vi "Read RawData.vi"(8 "error in (no error)":errorcluster, 9 "WCM":bool, 10 "# of scans":i32, 11 "UV-VIS in":refnum<class "CCD_camera.lvclass">) -> (0 "error out":errorcluster, 1 "Channel II OUT":sgl[][](array[numeric]), 2 "Channel I OUT":sgl[][](array[numeric]), 3 "UV-VIS out":refnum<class "CCD_camera.lvclass">, 4 "WCM_values OUT":sgl[](array[numeric]))   [LabVIEW 2015, in "CCD_camera.lvclass"]
uses:
  CCD_camera.lvclass
  dependecies/ControlsVIs/Clusters-def/Message types.ctl
  dependecies/ControlsVIs/Clusters-def/Standard Command.ctl
  dependecies/ControlsVIs/Clusters-def/OSc-WCM_max_value.ctl
  dependecies/Error Code Enum typedef.ctl
  Oscilloscope/Oscilloscope.lvclass
  Message/Message.lvclass
  GeneralFunctionality/GeneralFunctionality.lvclass
panel:
  in  "Booléen":bool
  out "error IO":errorcluster
  out "Graphe":i32[](graph)
  in  "Binning Horizontal":i32=1
  out "DLL error code":u32=20066
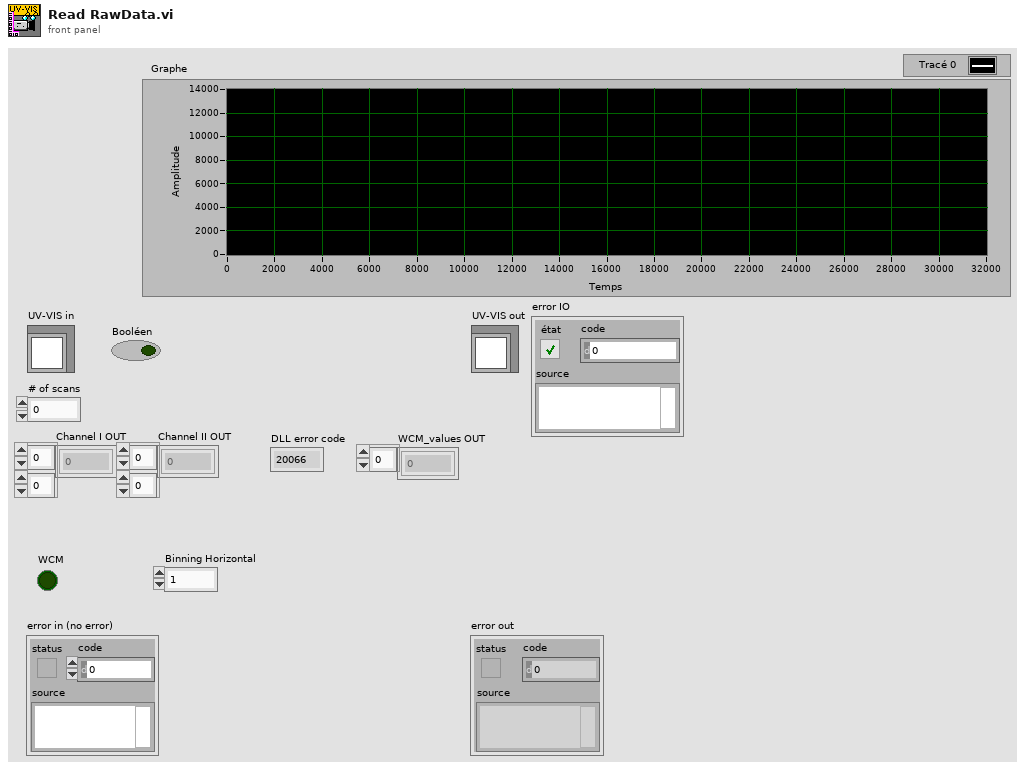
[diagram p1: front panel]
types:
  T1 = typedef "Message types.ctl" = string
  T2 = typedef "Standard Command.ctl" = cluster{"command":string, "data":variant}
  T3 = typedef "Oscilloscope.lvclass/OSc-WCM_max_value.ctl" = cluster{"WCM_max_value":dbl}
  T4 = typedef "Error Code Enum typedef.ctl" = enum32{"N/A (0)", "DRV_ERROR_CODES", "DRV_SUCCESS", "DRV_VXDNOTINSTALLED", "DRV_ERROR_SCAN", "DRV_ERROR_CHECK_SUM", "DRV_ERROR_FILELOAD", "DRV_UNKNOWN_FUNC", "DRV_ERROR_VXD_INIT", "DRV_ERROR_ADDRESS", "DRV_ERROR_PAGELOCK", "DRV_ERROR_PAGEUNLOCK", "DRV_ERROR_BOARDTEST", "DRV_ERROR_ACK", "DRV_ERROR_UP_FIFO", "DRV_ERROR_PATTERN", "N/A (16)", "DRV_ACQUISITION_ERRORS", "DRV_ACQ_BUFFER", "DRV_ACQ_DOWNFIFO_FULL", "DRV_PROC_UNKONWN_INSTRUCTION", "DRV_ILLEGAL_OP_CODE", "DRV_KINETIC_TIME_NOT_MET", "DRV_ACCUM_TIME_NOT_MET", "DRV_NO_NEW_DATA", "N/A (25)", "DRV_SPOOLERROR", "N/A (27)", "N/A (28)", "N/A (29)", "N/A (30)", "N/A (31)", "N/A (32)", "DRV_TEMPERATURE_CODES", "DRV_TEMPERATURE_OFF", "DRV_TEMPERATURE_NOT_STABILIZED", "DRV_TEMPERATURE_STABILIZED", "DRV_TEMPERATURE_NOT_REACHED", "DRV_TEMPERATURE_OUT_RANGE", "DRV_TEMPERATURE_NOT_SUPPORTED", "DRV_TEMPERATURE_DRIFT", "N/A (41)", "N/A (42)", "N/A (43)", "N/A (44)", "N/A (45)", "N/A (46)", "N/A (47)", "N/A (48)", "DRV_GENERAL_ERRORS", "DRV_INVALID_AUX", "DRV_COF_NOTLOADED", "DRV_FPGAPROG", "DRV_FLEXERROR", "DRV_GPIBERROR", "N/A (55)", "N/A (56)", "N/A (57)", "N/A (58)", "N/A (59)", "N/A (60)", "N/A (61)", "N/A (62)", "N/A (63)", "DRV_DATATYPE", "DRV_DRIVER_ERRORS", "DRV_P1INVALID", "DRV_P2INVALID", "DRV_P3INVALID", "DRV_P4INVALID", "DRV_INIERROR", "DRV_COFERROR", "DRV_ACQUIRING", "DRV_IDLE", "DRV_TEMPCYCLE", "DRV_NOT_INITIALIZED", "DRV_P5INVALID", "DRV_P6INVALID", "DRV_INVALID_MODE", "DRV_INVALID_FILTER", "DRV_I2CERRORS", "DRV_I2CDEVNOTFOUND", "DRV_I2CTIMEOUT", "DRV_P7INVALID", "N/A (84)", "N/A (85)", "N/A (86)", "N/A (87)", "N/A (88)", "N/A (89)", "DRV_IOCERROR", "DRV_VRMVERSIONERROR"}
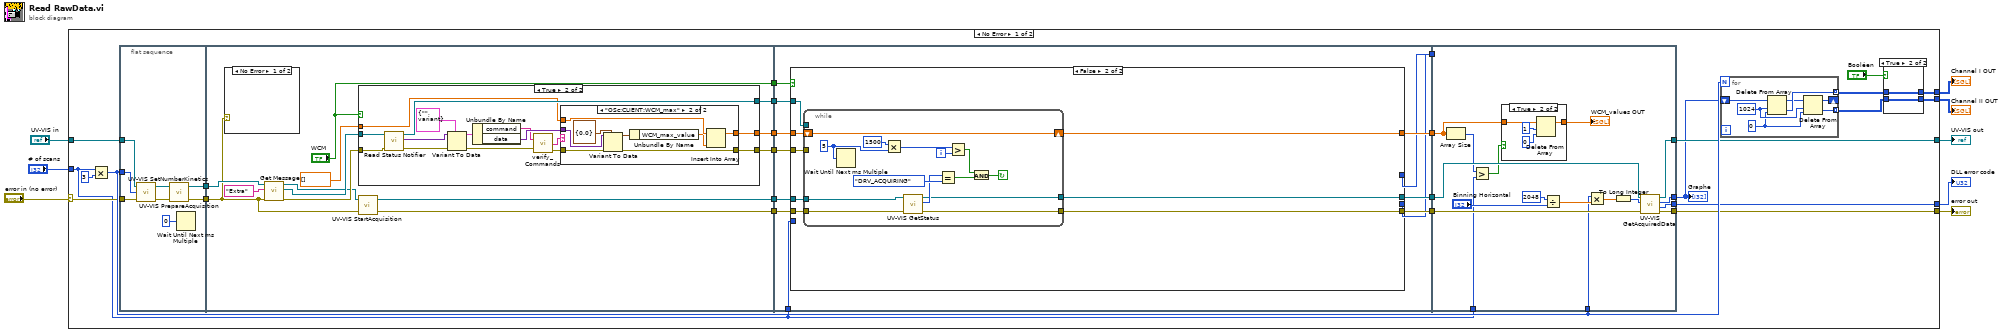
[diagram p0: block diagram]
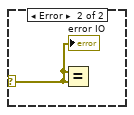
[diagram p3: hidden frame]
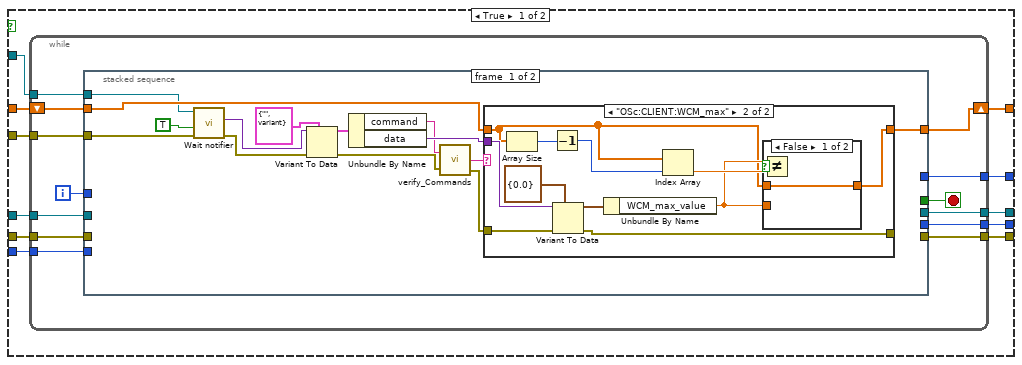
[diagram p6: hidden frame]
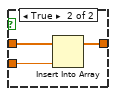
[diagram p8: hidden frame]
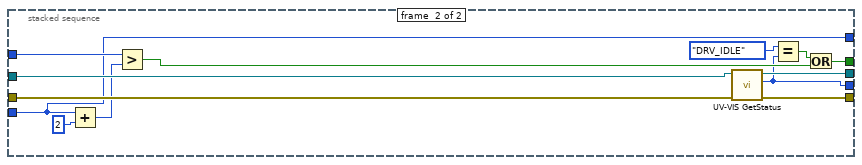
[diagram p9: hidden frame]
diagram:
  n1 = case shown="No Error" "error in (no error)" {
    selector: "error in (no error)" -> [w31 w223]
    tunnel: [w21 w223] -> w7
    tunnel: [w28 w222] -> w6
    tunnel: "UV-VIS in" -> [w30 w222]
    tunnel: "# of scans" -> [w16 _]
    tunnel: [w12 _] -> w3
    tunnel: [w11 _] -> w2
    tunnel: [w22 _] -> w1
    frame No Error {
      n2 = Multiply(x=w16, y=3) -> (x*y=w32:i32)
      n3 = flat-sequence {
        tunnel: [w52] -> w35
        tunnel: w32 -> [w51]
        tunnel: w30 -> [w49]
        tunnel: w31 -> [w50]
        tunnel: [w47] -> w29
        tunnel: w35 -> [w56]
        tunnel: [w67] -> w34
        tunnel: w29 -> [w65]
        tunnel: [w66] -> w27
        tunnel: ["WCM"] -> w24
        tunnel: [w61] -> w19
        tunnel: [w60] -> w18
        tunnel: [w59] -> w17
        tunnel: w34 -> [w108]
        tunnel: [w105] -> w26
        tunnel: w27 -> [w107]
        tunnel: [w106] -> w25
        tunnel: w24 -> [w100]
        tunnel: [w102] -> w23
        tunnel: w19 -> [w104]
        tunnel: w18 -> [w101]
        tunnel: w17 -> [w103]
        tunnel: w16 -> [w99]
        tunnel: [w98] -> w15
        tunnel: [w97] -> w14
        tunnel: w26 -> [w211]
        tunnel: w32 -> [w203]
        tunnel: w25 -> [w208]
        tunnel: [w215] -> w20
        tunnel: [w214] -> w22
        tunnel: [w209] -> w28
        tunnel: [w207] -> w21
        tunnel: w23 -> [w206]
        tunnel: w16 -> [w201]
        tunnel: w15 -> [_]
        tunnel: w14 -> [_]
        frame #0 {
          n4 = call "UV-VIS SetNumberKinetics.vi"("error in (no error)"=w50, "number"=w51, "Detector in"=w49) -> ("error out"=w54:errorcluster, "Detector out"=w48:refnum<class "CCD_camera.lvclass">)  [unwired: 1 out]
          n5 = call "UV-VIS PrepareAcquisition.vi"("error in (no error)"=w54, "Detector in"=w48) -> ("error out"=w52:errorcluster, "Detector out"=w47:refnum<class "CCD_camera.lvclass">)  [unwired: 1 in, 1 out]
          n6 = Wait Until Next ms Multiple(millisecond multiple=u32 0 ("n millisecondes")) -> ()  [unwired: 1 out]
        }
        frame #1 {
          n7 = case shown="No Error" w56 {
            selector: w56 -> [_ w68]
            frame No Error {
            }
            frame Error {
              n8 = Equal?(x=w68, y=w68) -> ()  [unwired: 1 out]
              "error IO" <- w68
            }
          }
          n9 = call "Get Message.vi"("error in (no error)"=w56, "Message type"=T1 "Extra", "GeneralFunctionality en entrée"=w65) -> ("error out"=w57:errorcluster, "Message.lvclass"=w58:refnum<class "Message.lvclass">, "GeneralFunctionality en sortie"=w55:refnum<class "CCD_camera.lvclass">)  [unwired: 6 in]
          n10 = case shown="True" "WCM" {
            tunnel: [w70 w72] -> w60
            tunnel: [w71 w86] -> w61
            tunnel: w58 -> [w71 w85]
            tunnel: w57 -> [w70 w81]
            tunnel: dbl[] [] -> [w69 w73]
            tunnel: [w69 w74] -> w59
            frame False {
            }
            frame True {
              n11 = call "Read Status Notifier.vi"("error in (no error)"=w81, "Message in"=w85) -> ("error out"=w80:errorcluster, "latest notification"=w82:variant, "Message out"=w86:refnum<class "Message.lvclass">)  [unwired: 6 in, 1 out]
              n12 = Variant To Data(error in=w80, type=T2 {"command"="", "data"=variant} ("input cluster"), Variant=w82) -> (data=w84:T2, error out=w75:errorcluster)
              n13 = Unbundle By Name(w84) -> ("command"=w76:string, "data"=w79:variant)
              n14 = call "verify_Commands.vi"("Command"=w76, "error in"=w75) -> ("Command out"=w77:string, "error out"=w78:errorcluster)  [unwired: 1 out]
              n15 = case shown="\"OSc:CLIENT:WCM_max\"" w77 {
                tunnel: w78 -> [w88 w96]
                tunnel: [w88 w94] -> w72
                tunnel: w79 -> [_ w95]
                tunnel: w73 -> [w87 w91]
                tunnel: [w87 w90] -> w74
                frame "Error", Default {
                }
                frame "OSc:CLIENT:WCM_max" {
                  n16 = Variant To Data(error in=w96, type=T3 {"WCM_max_value"=0.0} ("ELYSE pulses counter"), Variant=w95) -> (data=w92:T3, error out=w94:errorcluster)
                  n17 = Unbundle By Name(w92) -> ("WCM_max_value"=w89:dbl)
                  n18 = Insert Into Array(array=w91, new element=w89) -> (w90:dbl[])  [unwired: 1 in]
                }
              }
            }
          }
          n19 = call "UV-VIS StartAcquisition.vi"("error in (no error)"=w56, "Detector in"=w55) -> ("error out"=w67:errorcluster, "Detector out"=w66:refnum<class "CCD_camera.lvclass">)  [unwired: 1 in, 1 out]
        }
        frame #2 {
          n20 = case shown="False" w100 {
            tunnel: w108 -> [w119 w185]
            tunnel: w107 -> [w118 w184]
            tunnel: [w113 w183] -> w106
            tunnel: [w112 w182] -> w105
            tunnel: w104 -> [w117 w181]
            tunnel: w103 -> [w116 w180]
            tunnel: [w115 w179] -> w102
            tunnel: w101 -> [w114 w178]
            tunnel: w99 -> [w111 _]
            tunnel: [w110 _] -> w98
            tunnel: [w109 _] -> w97
            frame True {
              n21 = while {
                tunnel: w119 -> [w127]
                tunnel: w118 -> [w128]
                tunnel: w117 -> [w130]
                shift-right: [w131] -> w115
                shift-left: w116 -> [w132]
                tunnel: w114 -> [w129]
                tunnel: [w126] -> w113
                tunnel: [w125] -> w112
                tunnel: w111 -> [w122]
                tunnel: [w121] -> w110
                tunnel: [w120] -> w109
                i -> [w124]
                stop <- w123 stop-if-true
                n22 = stacked-sequence {
                  tunnel: w132 -> [w146 _]
                  tunnel: [w145 _] -> w131
                  tunnel: w130 -> [w137 _]
                  tunnel: w129 -> [w136 _]
                  tunnel: w128 -> [_ w177]
                  tunnel: w127 -> [_ w175]
                  tunnel: [_ w176] -> w126
                  tunnel: [_ w174] -> w125
                  tunnel: w124 -> [_ w170]
                  tunnel: [_ w169] -> w123
                  tunnel: w122 -> [_ w165]
                  tunnel: [_ w166] -> w121
                  tunnel: [_ w165] -> w120
                  frame #0 {
                    n23 = call "Wait notifier.vi"("error in (no error)"=w136, "ignorer les précédents (F)"=TRUE, "Message en entrée"=w137) -> ("error out"=w134:errorcluster, "notification"=w135:variant)  [unwired: 6 in, 1 out]
                    n24 = Variant To Data(error in=w134, type=T2 {"command"="", "data"=variant} ("input cluster"), Variant=w135) -> (data=w144:T2, error out=w138:errorcluster)
                    n25 = Unbundle By Name(w144) -> ("command"=w139:string, "data"=w142:variant)
                    n26 = call "verify_Commands.vi"("Command"=w139, "error in"=w138) -> ("Command out"=w140:string, "error out"=w141:errorcluster)  [unwired: 1 out]
                    n27 = case shown="\"OSc:CLIENT:WCM_max\"" w140 {
                      tunnel: w141 -> [w148 w160]
                      tunnel: [w148 w158] -> _
                      tunnel: w142 -> [_ w159]
                      tunnel: w146 -> [w147 w151]
                      tunnel: [w147 w155] -> w145
                      frame "Error", Default {
                      }
                      frame "OSc:CLIENT:WCM_max" {
                        n28 = Array Size(array=w151) -> (size(s)=w150:i32)
                        n29 = Decrement(x=w150) -> (x-1=w149:i32)
                        n30 = Variant To Data(error in=w160, type=T3 {"WCM_max_value"=0.0} ("ELYSE pulses counter"), Variant=w159) -> (data=w156:T3, error out=w158:errorcluster)
                        n31 = Unbundle By Name(w156) -> ("WCM_max_value"=w152:dbl)
                        n32 = Index Array(array=w151, index=w149) -> (element=w154:dbl)
                        n33 = Not Equal?(x=w152, y=w154) -> (x != y?=w153:bool)
                        n34 = case shown="False" w153 {
                          tunnel: w151 -> [w161 w164]
                          tunnel: [w161 w163] -> w155
                          tunnel: w152 -> [_ w162]
                          frame False {
                          }
                          frame True {
                            n35 = Insert Into Array(array=w164, new element=w162) -> (w163:dbl[])  [unwired: 1 in]
                          }
                        }
                      }
                    }
                  }
                  frame #1 {
                    n36 = Add(x=w165, y=2) -> (x+y=w168:i32)
                    n37 = Greater?(x=w170, y=w168) -> (0:w171:bool)
                    n38 = call "UV-VIS GetStatus.vi"("error in (no error)"=w175, "Detector in"=w177) -> ("error out"=w174:errorcluster, "status"=w166:T4, "Detector out"=w176:refnum<class "CCD_camera.lvclass">)  [unwired: 2 in, 1 out]
                    n39 = Equal?(x=Error_Code_Enum_typedef."DRV_IDLE" ("y"), y=w166) -> (x = y?=w172:bool)
                    n40 = Or(x=w172, y=w171) -> (x .or. y?=w169:bool)
                  }
                }
              }
            }
            frame False {
              n41 = while {
                tunnel: w185 -> [w197]
                tunnel: [w196] -> w182
                tunnel: w184 -> [w195]
                tunnel: [w194] -> w183
                tunnel: w181 -> [_]
                shift-right: [w186] -> w179
                shift-left: w180 -> [w186]
                tunnel: w178 -> [_]
                i -> [w187]
                stop <- w191 continue-if-true
                w189 = u32 5 ("n millisecondes")
                n42 = Wait Until Next ms Multiple(millisecond multiple=w189) -> ()  [unwired: 1 out]
                n43 = Multiply(x=1500 ("y"), y=w189) -> (x*y=w188:u32)
                n44 = call "UV-VIS GetStatus.vi"("error in (no error)"=w197, "Detector in"=w195) -> ("error out"=w196:errorcluster, "status"=w198:T4, "Detector out"=w194:refnum<class "CCD_camera.lvclass">)  [unwired: 2 in, 1 out]
                n45 = Equal?(x=w198, y=Error_Code_Enum_typedef."DRV_ACQUIRING") -> (x = y?=w193:bool)
                n46 = Greater?(x=w188, y=w187) -> (0:w192:bool)
                n47 = And(x=w192, y=w193) -> (x .and. y?=w191:bool)
              }
            }
          }
        }
        frame #3 {
          n48 = Array Size(array=w206) -> (size(s)=w204:i32)
          n49 = Greater?(x=w204, y=w201) -> (0:w205:bool)
          n50 = case shown="True" w205 {
            tunnel: [w217 w219] -> w202
            tunnel: w206 -> [w217 w221]
            frame False {
            }
            frame True {
              n51 = Delete From Array(array=w221, length=1, index=0) -> (array with subset deleted=w219:dbl[])  [unwired: 1 out]
            }
          }
          "WCM_values OUT" <- w202
          n52 = Divide(x=2048 ("y"), y="Binning Horizontal") -> (x/y=w213:dbl)
          n53 = Multiply(x=w203, y=w213) -> (x*y=w216:dbl)
          n54 = To Long Integer(number=w216) -> (32bit integer=w200:i32)
          n55 = call "UV-VIS GetAcquiredData.vi"("error in (no error)"=w211, "size"=w200, "Detector in"=w208) -> ("error out"=w207:errorcluster, "DLL error code"=w214:u32, "array"=w215:i32[], "Detector out"=w209:refnum<class "CCD_camera.lvclass">)  [unwired: 1 in]
        }
      }
      n56 = for {
        N: w32 -> [_]
        shift-right: [w40] -> _
        shift-left: w20 -> [w46]
        tunnel: [w45] -> w10 mode=indexing
        tunnel: [w41] -> w9 mode=indexing
        w42 = 0 ("index")
        w43 = 1024 ("length")
        n57 = Delete From Array(array=w46, length=w43, index=w42) -> (deleted portion=w45:i32[], array with subset deleted=w44:i32[])
        n58 = Delete From Array(array=w44, length=w43, index=w42) -> (deleted portion=w41:i32[], array with subset deleted=w40:i32[])
      }
      n59 = case shown="True" "Booléen" {
        tunnel: [w36 w39] -> w12
        tunnel: w10 -> [w37 w39]
        tunnel: w9 -> [w36 w38]
        tunnel: [w37 w38] -> w11
        frame False {
        }
        frame True {
        }
      }
      "Graphe" <- w20
    }
    frame Error {
    }
  }
  "error out" <- w7
  "UV-VIS out" <- w6
  "Channel I OUT" <- w3
  "Channel II OUT" <- w2
  "DLL error code" <- w1
